vi "DCMotor_GetCurrent.vi"(9 "VoltageInput_Volts":dbl format="%13.5p", 10 "Speed_RadPerSec":dbl format="%13.5p", 11 "DCMOTOR":T1 {"Kt_NMPerAmp" format="%13.5p"; "Kv_RadPerSecPerVolt" format="%13.5p"; "R_Ohms" format="%13.5p"; "FreeSpeed_RadPerSec" format="%13.5p"; "FreeCurrent_Amps" format="%13.5p"; "StallCurrent_Amps" format="%13.5p"; "StallTorque_NM" format="%13.5p"; "nominalVoltage_Volts" format="%13.5p"}) -> (3 "Current_Amps":dbl format="%13.5p")   [LabVIEW 2019, in "Trajectory_Library.lvlib"]
doc: "Estimates DC Motor current.\n\n\nInputs: \n - XXX -- XXX.\n\nOutputs:\n - XXX -- XXX."
uses:
  Trajectory_Library.lvlib
  DCMOTOR.CTL
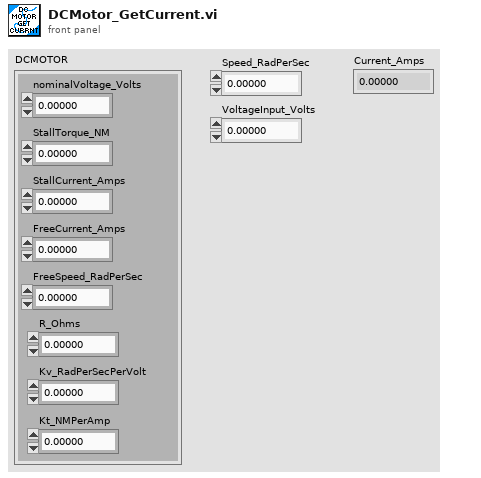
[diagram p1: front panel]
types:
  T1 = typedef "Trajectory_Library.lvlib/DCMOTOR.CTL" = cluster{"nominalVoltage_Volts":dbl, "StallTorque_NM":dbl, "StallCurrent_Amps":dbl, "FreeCurrent_Amps":dbl, "FreeSpeed_RadPerSec":dbl, "R_Ohms":dbl, "Kv_RadPerSecPerVolt":dbl, "Kt_NMPerAmp":dbl}
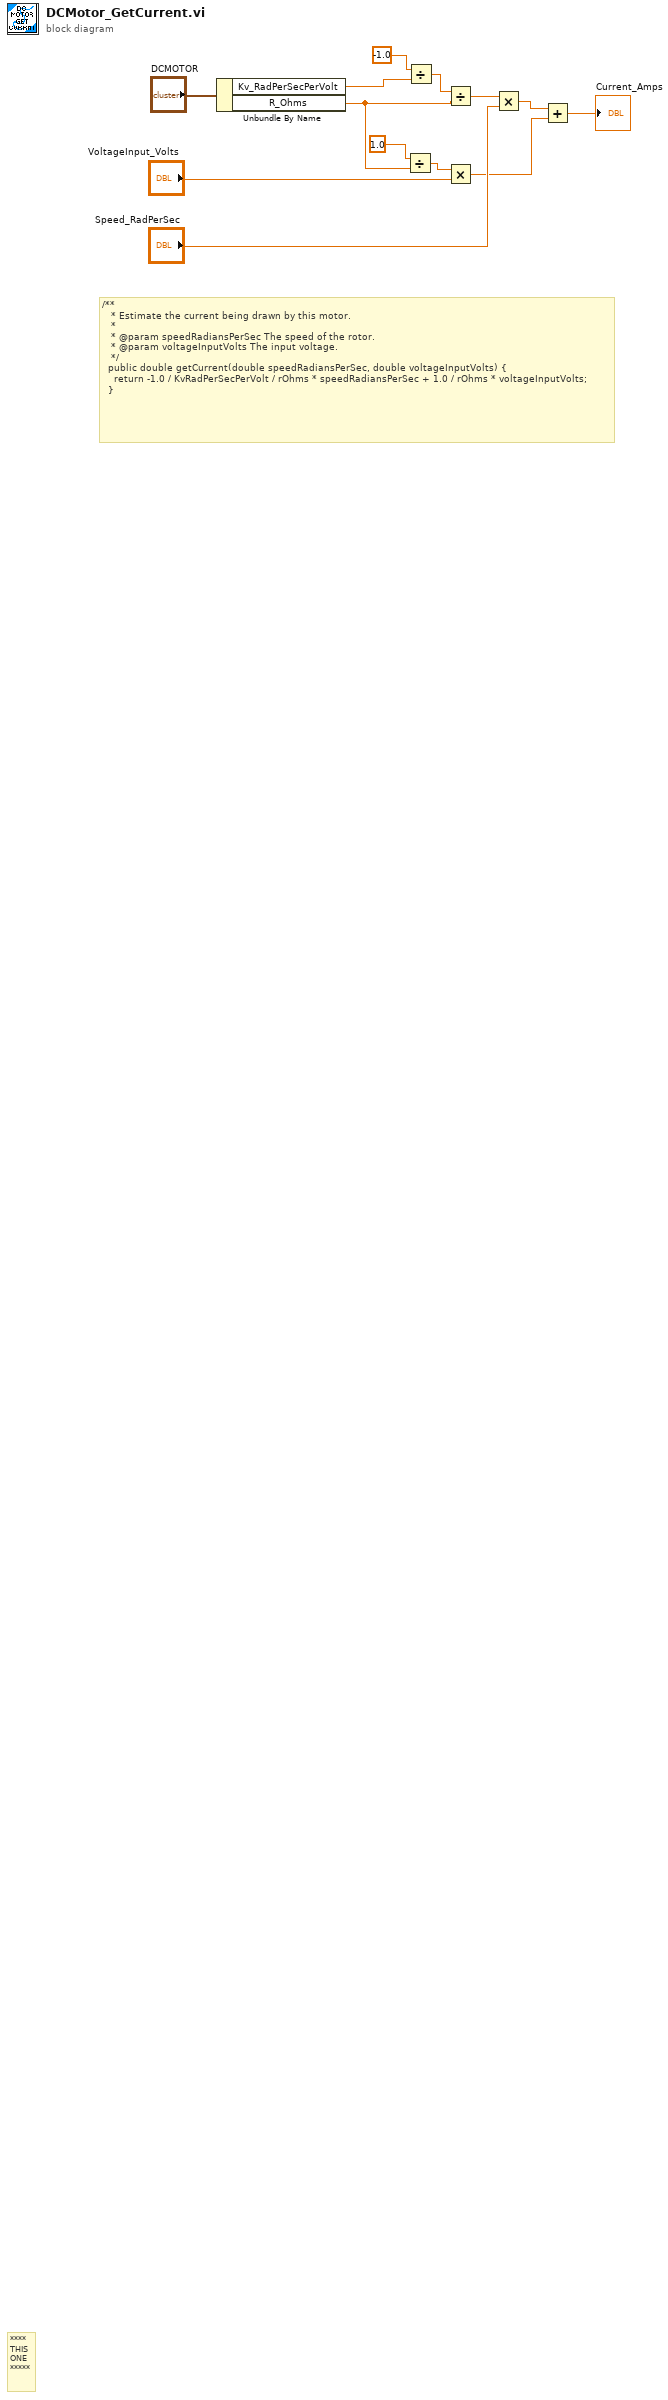
[diagram p0: block diagram]
diagram:
  # "/**\n   * Estimate the current being drawn by this motor.\n   *\n   * @param speedRadiansPerSec The speed of the rotor.\n   * @param voltageInputVolts The input voltage.\n   */\n  public double getCurrent(double speedRadiansPerSec, double voltageInputVolts) {\n    return -1.0 / KvRadPerSecPerVolt / rOhms * speedRadiansPerSec + 1.0 / rOhms * voltageInputVolts;\n  }"
  # "****\nTHIS\nONE\n*****"
  n1 = Unbundle By Name("DCMOTOR") -> ("Kv_RadPerSecPerVolt"=w11:dbl, "R_Ohms"=w5:dbl)
  n2 = Divide(x=1.0, y=w5) -> (x/y=w6:dbl)
  n3 = Divide(x=-1.0, y=w11) -> (x/y=w10:dbl)
  n4 = Divide(x=w10, y=w5) -> (x/y=w8:dbl)
  n5 = Multiply(x=w6, y="VoltageInput_Volts") -> (x*y=w2:dbl)
  n6 = Multiply(x=w8, y="Speed_RadPerSec") -> (x*y=w3:dbl)
  n7 = Add(x=w3, y=w2) -> (x+y=→"Current_Amps":dbl)
